vi "Do I Downshift.vi"(8 "Cluster":T1) -> (5 "Enum":T3)   [LabVIEW 2013]
uses:
  Drive Train States.ctl
  Drive Train Metrics.ctl
  CmdFlag.ctl
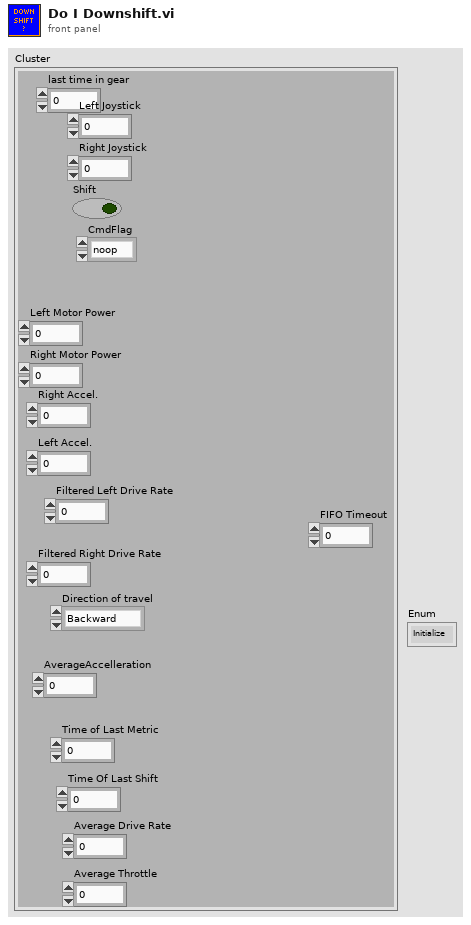
[diagram p1: front panel]
types:
  T1 = typedef "Drive Train Metrics.ctl" = cluster{"last time in gear":u32, "Shift":bool, "Right Joystick":dbl, "Left Joystick":dbl, "CmdFlag":T2, "Right Motor Power":dbl, "Left Motor Power":dbl, "Right Accel.":dbl, "Left Accel.":dbl, "Filtered Left Drive Rate":dbl, "Filtered Right Drive Rate":dbl, "Direction of travel":enum16{"Backward", "Forward", "Spin"}, "AverageAccelleration":dbl, "Time of Last Metric":u32, "Time Of Last Shift":dbl, "Average Drive Rate":dbl, "Average Throttle":dbl, "FIFO Timeout":i32}
  T2 = typedef "CmdFlag.ctl" = enum16{"noop", "suspend", "resume"}
  T3 = typedef "Drive Train States.ctl" = enum16{"Initialize", "Low_gear", "Upshift", "Wait For Upshift", "Upshift Complete", "High_gear", "Downshift", "Wait For Downshift", "Downshift Complete", "Suspend", "Resume"}
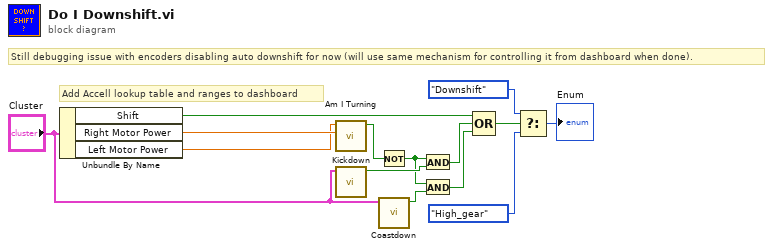
[diagram p0: block diagram]
diagram:
  # "Add Accell lookup table and ranges to dashboard"
  # "Still debugging issue with encoders disabling auto downshift for now (will use same mechanism for controlling it from dashboard when done)."
  n1 = Unbundle By Name("Cluster") -> ("Shift"=w11:bool, "Right Motor Power"=w9:dbl, "Left Motor Power"=w8:dbl)
  n2 = call "Am I Turning.vi"("Right Joystick"=w9, "Left Joystick"=w8) -> ("Turn?"=w5:bool)  [unwired: 9 in]
  n3 = call "Kickdown.vi"("Cluster"="Cluster") -> ("Shift?"=w6:bool)  [unwired: 10 in]
  n4 = Not(x=w5) -> (.not. x?=w4:bool)
  n5 = call "Coastdown.vi"("Cluster"="Cluster") -> ("Boolean"=w2:bool)  [unwired: 10 in]
  n6 = And(x=w4, y=w6) -> (x .and. y?=w7:bool)
  n7 = And(x=w4, y=w2) -> (x .and. y?=w1:bool)
  n8 = Compound Arithmetic op=OR(w11, w7, w1) -> (w10:bool)
  n9 = Select(t=Drive_Train_States."Downshift", s=w10, f=Drive_Train_States."High_gear") -> (s? t:f=→"Enum":T3)
